vi "Check Touch Setting).vi"(8 "error in (no error)":errorcluster) -> (0 "error out":errorcluster, 3 "Boolean":bool)   [LabVIEW 2017]
uses:
  <vilib>/registry/registry.llb/Registry RtKey.ctl
  <vilib>/registry/registry.llb/Registry SAM.ctl
  <vilib>/registry/registry.llb/Registry View.ctl
  <vilib>/registry/registry.llb/Read Registry Value Simple STR.vi
panel:
  out "String/Binary data":string
  out "simple data type":enum16{"String", "Binary", "DWORD"}(ring)
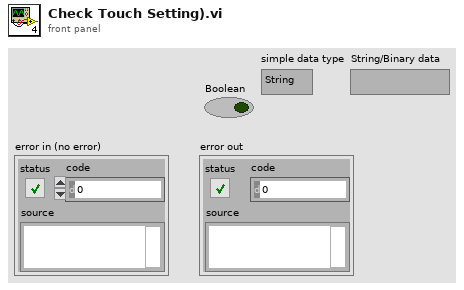
[diagram p1: front panel]
types:
  T1 = typedef "Registry View.ctl" = u16
  T2 = typedef "Registry SAM.ctl" = enum32{"KEY_QUERY_VALUE", "KEY_SET_VALUE", "KEY_CREATE_SUB_KEY", "KEY_ENUMERATE_SUB_KEYS", "KEY_NOTIFY", "KEY_CREATE_LINK", "KEY_READ", "KEY_WRITE", "KEY_ALL_ACCESS", "KEY_READ | KEY_WRITE"}
  T3 = typedef "Registry RtKey.ctl" = enum32{"HKEY_CLASSES_ROOT", "HKEY_CURRENT_USER", "HKEY_LOCAL_MACHINE", "HKEY_USERS", "HKEY_PERFORMANCE_DATA", "HKEY_CURRENT_CONFIG", "HKEY_DYN_DATA"}
  T4 = typedef "Registry refnum.ctl" = refnum<k1>
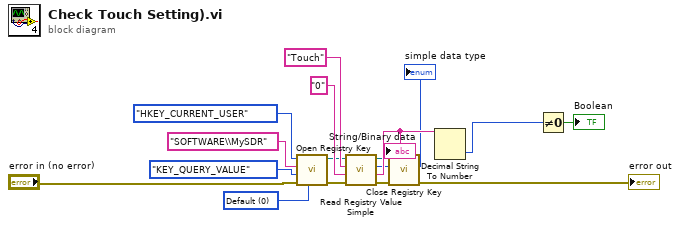
[diagram p0: block diagram]
diagram:
  w7 = T1 0 items=["Default"=0, "KEY_WOW64_64KEY"=8, "KEY_WOW64_32KEY"=9] ("registry view")
  n1 = call <vilib>:"Open Registry Key.vi"("registry view"=w7, "error in (no error)"="error in (no error)", "security access mask (KEY_READ | KEY_WRITE)"=Registry_SAM."KEY_QUERY_VALUE", "subkey"="SOFTWARE\\MySDR", "root key (HKEY_LOCAL_MACHINE)"=Registry_RtKey."HKEY_CURRENT_USER") -> ("error out"=w9:errorcluster, "refnum out"=w6:T4)  [unwired: 5 in]
  n2 = call-poly <vilib>:"Read Registry Value Simple.vi"("error in (no error)"=w9, "default data"="0", "value"="Touch", "refnum"=w6) -> ("error out"=w10:errorcluster, "String/Binary data"=w16:string, "simple data type"=→"simple data type":enum16{"String", "Binary", "DWORD"}, "refnum out"=w11:T4)  [unwired: 2 in]
  "String/Binary data" <- w16
  n3 = call <vilib>:"Close Registry Key.vi"("error in (no error)"=w10, "refnum"=w11) -> ("error out"=→"error out":errorcluster)  [unwired: 5 in]
  n4 = Decimal String To Number(string=w16) -> (number=w1:i32)  [unwired: 2 in, 1 out]
  n5 = Not Equal To 0?(x=w1) -> (x != 0?=→"Boolean":bool)
